vi "Toggle-pane.vi"(8 "error in (no error)":errorcluster, 10 "Pane":T1, 11 "Panes in":T2) -> (0 "error out":errorcluster, 2 "Status":bool, 3 "Panes out":T2)   [LabVIEW 2013, in "HardwareCharacterization.lvlib" / "HC-UI.lvclass"]
uses:
  HC-UI.lvclass
  Panes-reference.ctl
  Pane-names.ctl
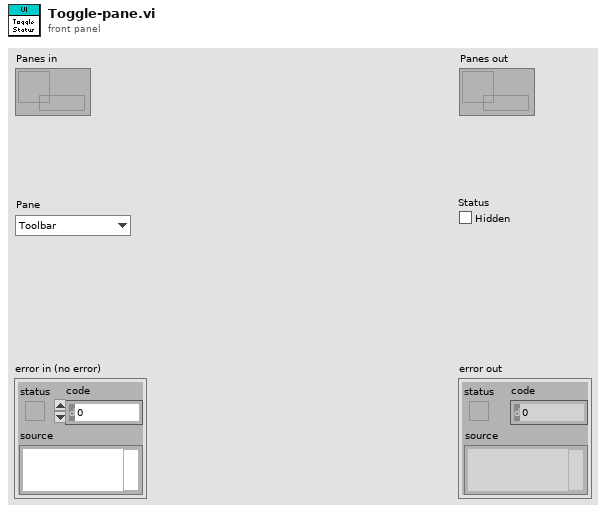
[diagram p1: front panel]
types:
  T1 = typedef "HardwareCharacterization.lvlib/HC-UI.lvclass/Pane-names.ctl" = enum16{"Toolbar", "Help bar", "Toolbar lower border", "Center panel", "Main panel", "Settings panel", "Status bar upper border", "General state bar", "Information bar"}
  T2 = typedef "HardwareCharacterization.lvlib/HC-UI.lvclass/Panes-reference.ctl" = refnum<data-value>
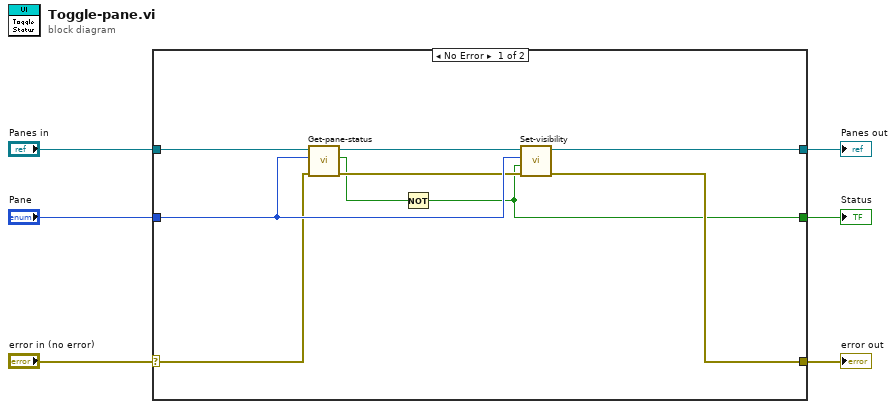
[diagram p0: block diagram]
diagram:
  n1 = case shown="No Error" "error in (no error)" {
    selector: "error in (no error)" -> [w10 w16]
    tunnel: [w13 w16] -> w5
    tunnel: [w14 w17] -> w3
    tunnel: "Panes in" -> [w15 w17]
    tunnel: "Pane" -> [w11 _]
    tunnel: [w7 _] -> w1
    frame No Error {
      n2 = call "Get-pane-status.vi"("error in (no error)"=w10, "Pane"=w11, "Panes in"=w15) -> ("error out"=w9:errorcluster, "Status"=w8:bool, "Panes out"=w12:T2)  [unwired: 6 in]
      n3 = Not(x=w8) -> (.not. x?=w7:bool)
      n4 = call "Set-visibility.vi"("error in (no error)"=w9, "Visibility"=w7, "Pane"=w11, "Panes in"=w12) -> ("error out"=w13:errorcluster, "Panes out"=w14:T2)  [unwired: 6 in]
    }
    frame Error {
    }
  }
  "error out" <- w5
  "Panes out" <- w3
  "Status" <- w1
